vi "PATCH.vi"(6 "timeout":i32=10000, 7 "output file":path, 8 "error in":errorcluster, 9 "buffer":string, 10 "url":string, 11 "http-client in":refnum<class "http-method-patch.lvclass">) -> (0 "error out":errorcluster, 1 "body":string, 2 "headers":string, 3 "http-client out":refnum<class "http-method-patch.lvclass">)   [LabVIEW 2020, in "REST Client.lvlib" / "http-method-patch.lvclass"]
uses:
  http-method-patch.lvclass
  http-client/http-client.lvclass
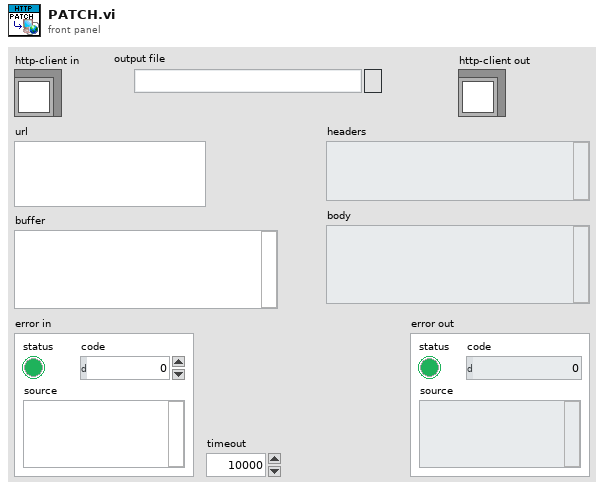
[diagram p1: front panel]
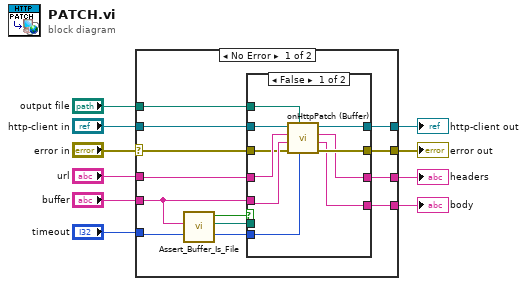
[diagram p0: block diagram]
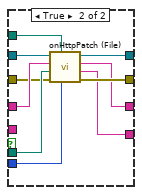
[diagram p2: hidden frame]
diagram:
  n1 = case shown="No Error" "error in" {
    selector: "error in" -> [w11 w44]
    tunnel: [w12 w44] -> w9
    tunnel: [w17 w43] -> w7
    tunnel: "http-client in" -> [w19 w43]
    tunnel: [w16 _] -> w6
    tunnel: "url" -> [w13 _]
    tunnel: "timeout" -> [w14 _]
    tunnel: "output file" -> [w18 _]
    tunnel: [w15 _] -> w2
    tunnel: "buffer" -> [w20 _]
    frame No Error {
      n2 = call "Assert_Buffer_Is_File.vi"("body"=w20) -> ("File"=w21:path, "is File?"=w22:bool)  [unwired: 9 in]
      n3 = case shown="False" w22 {
        tunnel: w21 -> [_ w39]
        tunnel: w20 -> [w25 _]
        tunnel: w19 -> [w23 w41]
        tunnel: w18 -> [w31 w42]
        tunnel: [w32 w33] -> w17
        tunnel: [w27 w34] -> w16
        tunnel: [w28 w35] -> w15
        tunnel: w14 -> [w30 w38]
        tunnel: w13 -> [w26 w40]
        tunnel: [w29 w36] -> w12
        tunnel: w11 -> [w24 w37]
        frame False {
          n4 = call-dynamic "onHttpPatch (Buffer).vi"("timeout"=w30, "output file"=w31, "error in"=w24, "buffer"=w25, "url"=w26, "http-client in"=w23) -> ("error out"=w29:errorcluster, "body"=w28:string, "headers"=w27:string, "http-client out"=w32:refnum<class "http-method-patch.lvclass">)  [unwired: 2 in]
        }
        frame True {
          n5 = call-dynamic "onHttpPatch (File).vi"("timeout"=w38, "output file"=w42, "error in"=w37, "file"=w39, "url"=w40, "http-client in"=w41) -> ("error out"=w36:errorcluster, "body"=w35:string, "headers"=w34:string, "http-client out"=w33:refnum<class "http-method-patch.lvclass">)  [unwired: 2 in]
        }
      }
    }
    frame Error {
    }
  }
  "error out" <- w9
  "http-client out" <- w7
  "headers" <- w6
  "body" <- w2
